vi "GyroFSRangeToDouble.vi"(11 "GyroFSRange":T1) -> (3 "Double":dbl)   [LabVIEW 2016]
uses:
  GyroFSRange.ctl
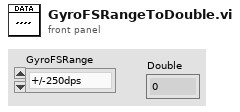
[diagram p1: front panel]
types:
  T1 = typedef "GyroFSRange.ctl" = enum16{"+/-250dps", "+/-500dps", "+/-1000dps", "+/-2000dps"}
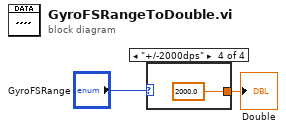
[diagram p0: block diagram]
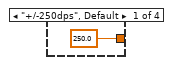
[diagram p2: hidden frame]
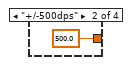
[diagram p3: hidden frame]
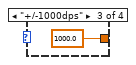
[diagram p4: hidden frame]
diagram:
  n1 = case shown="\"+/-2000dps\"" "GyroFSRange" {
    tunnel: [250.0 500.0 1000.0 2000.0] -> w1
    frame "+/-250dps", Default {
    }
    frame "+/-500dps" {
    }
    frame "+/-1000dps" {
    }
    frame "+/-2000dps" {
    }
  }
  "Double" <- w1
